vi "Main_old.vi"() -> ()   [LabVIEW 2020]
uses:
  States.ctl
  <vilib>/Instr/_visa.llb/VISA Configure Serial Port (Serial Instr).vi
  <vilib>/Utility/file.llb/Read Delimited Spreadsheet (I64).vi
panel:
  out "Last Inc Sent":string
  out "Last Speed Sent":string
  out "Next Control State":T1
  out "Next Com State":enum16{"Initialize", "Send", "Receive", "Error"}(ring)=enum."Receive"
  out "Next Cmd":enum16{"getParm", "inc", "mph", "err"}(ring)
  out "Send Buffer":string
  out "Control Error":errorcluster
  out "Com Error":errorcluster
  out "Missed Msg":u16
  out "Time Left":u32
  out "Inc Changed":bool
  out "Next MPH":u16
  out "Next Duration":u16
  out "Next Inc":u16
  out "PD READ":u8
  out "INC READ":u8
  out "MPH READ":u8
  out "dwell":u16[](array[numeric])
  out "incline":u16[](array[numeric])
  out "time":u16[](array[numeric])
  out "speed":u16[](array[numeric])
  out "input lines":i32
  in  "TestScript":path=path "C:/LabView Computer Backup SEAL2788/DonP_TRM500/FootTimeInc.txt"
  out "read buffer":string
  out "Speed Changed":bool
  in  "Manual Stop":bool
  in  "Serial Port":refnum<visa-resource-name>="COM8"
  out "FootPath":path
  out "FootPathRef":refnum<file>
  out "stopping":bool
  out "Target MPH":u16 max=12 step=1
  out "step":i32
  out "Target INC":u16 max=12 step=1
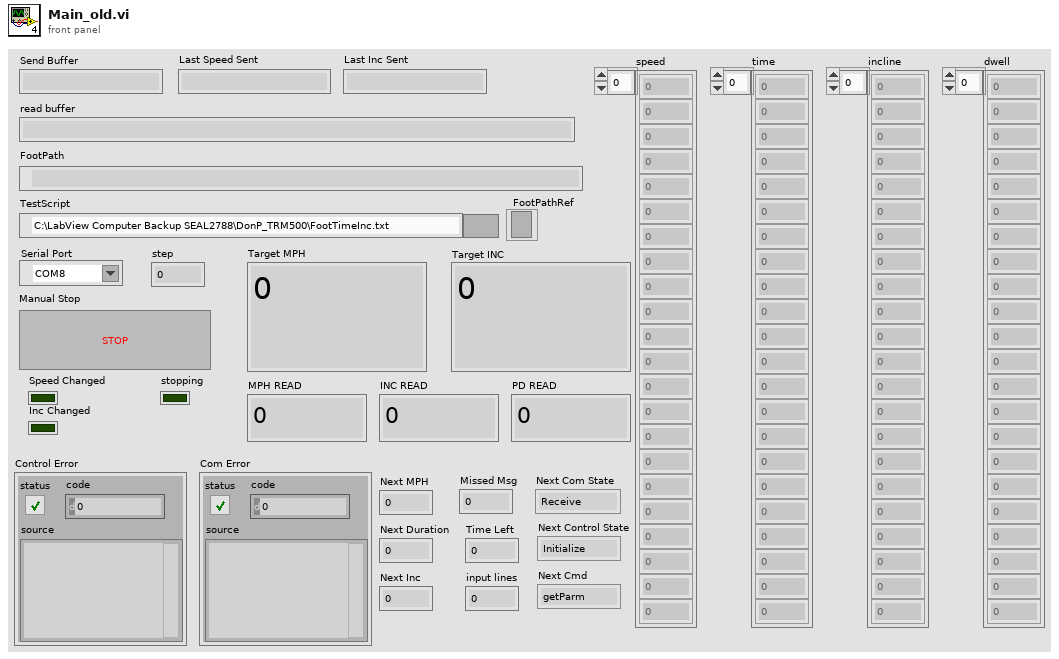
[diagram p1: front panel]
types:
  T1 = typedef "States.ctl" = enum16{"Initialize", "SetTargets", "WaitforMPH", "Dwell", "CheckTiming"}
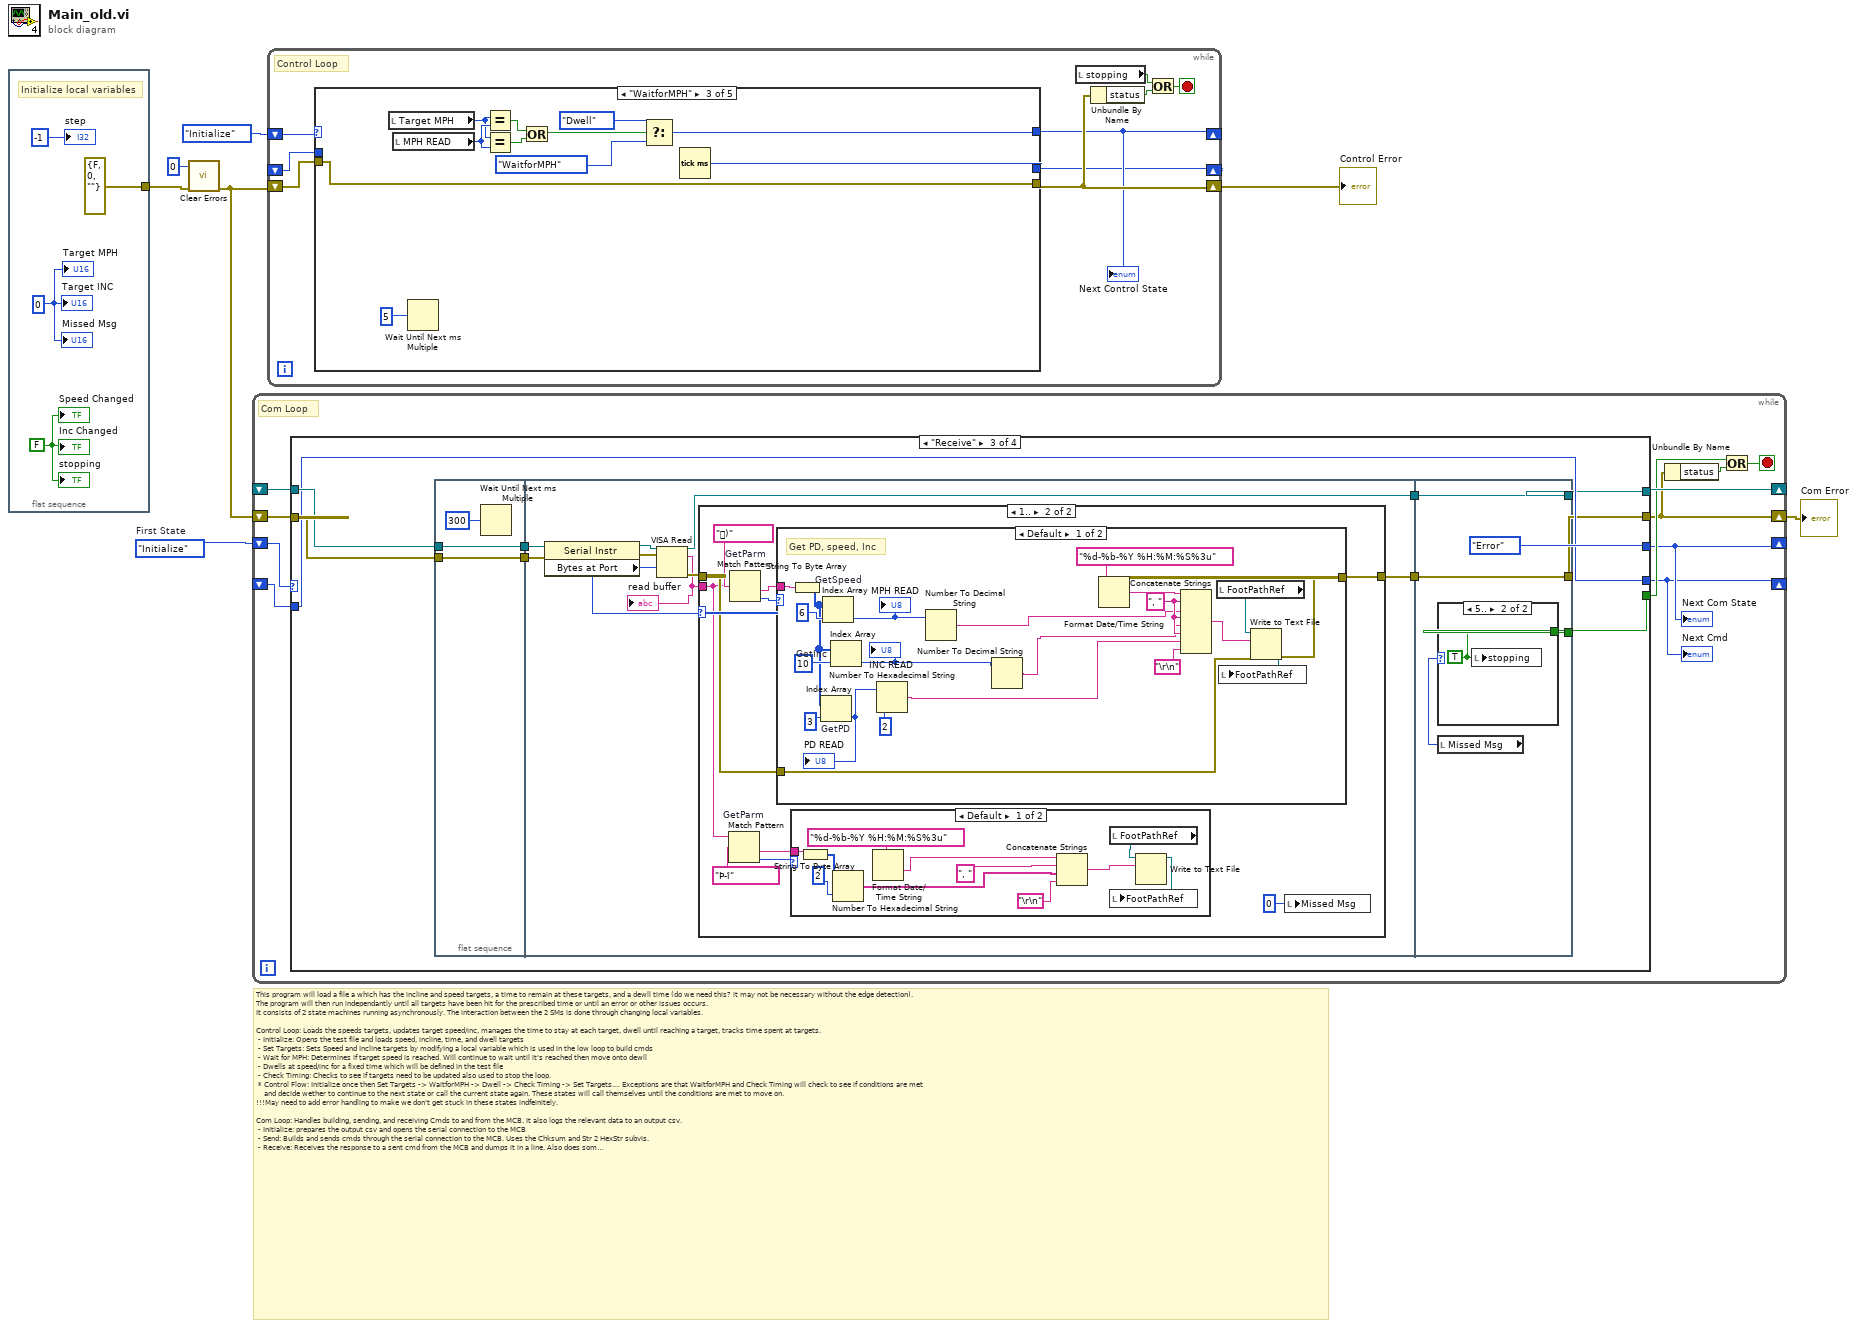
[diagram p0: block diagram]
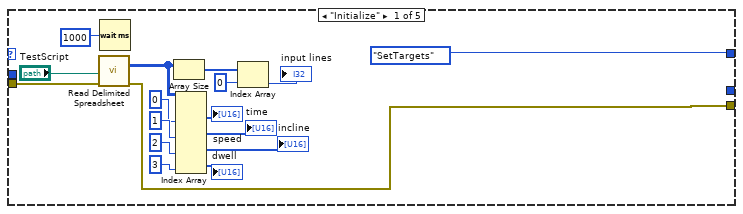
[diagram p2: hidden frame]
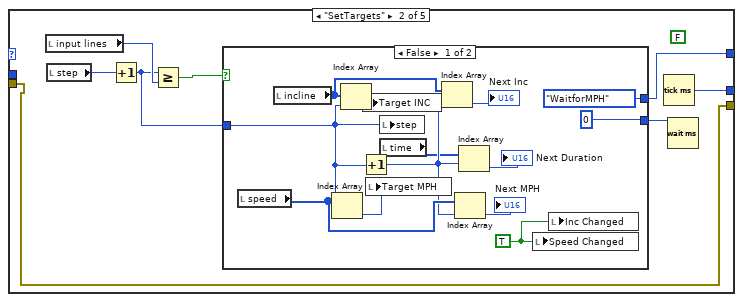
[diagram p3: hidden frame]
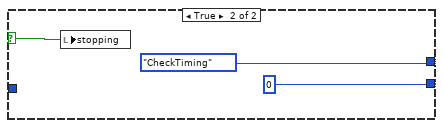
[diagram p4: hidden frame]
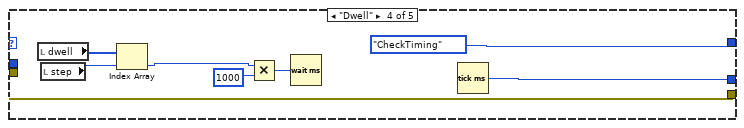
[diagram p5: hidden frame]
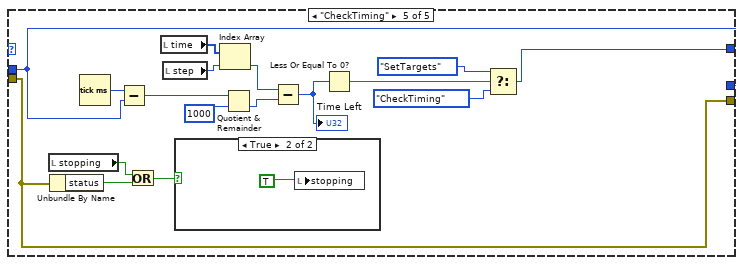
[diagram p6: hidden frame]
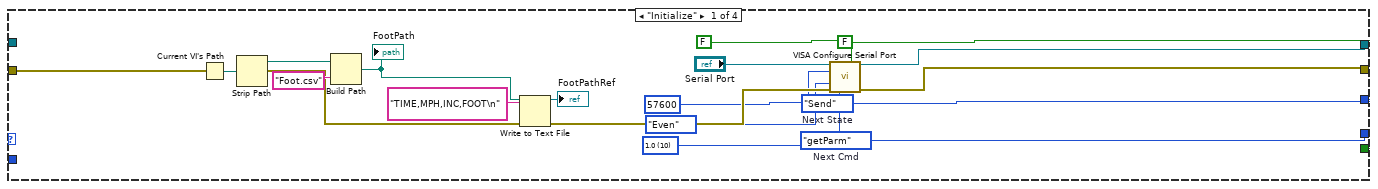
[diagram p8: hidden frame]
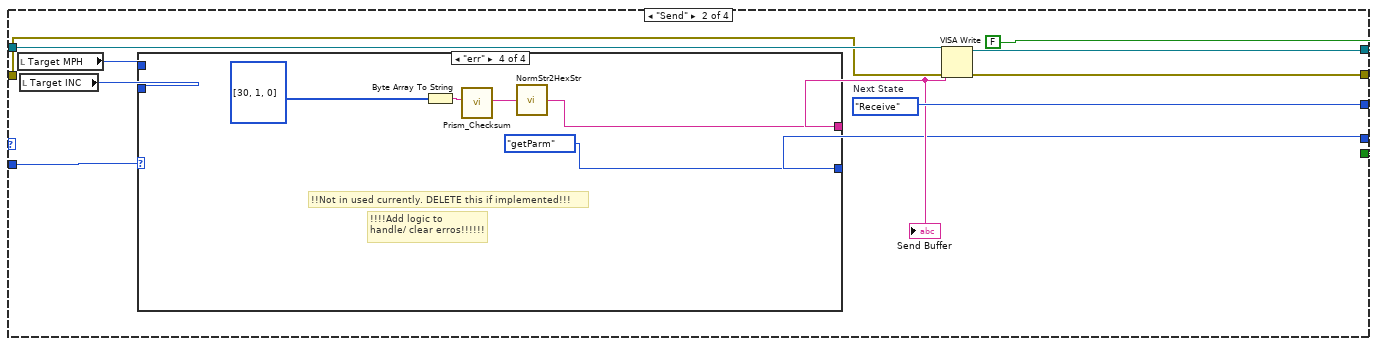
[diagram p9: hidden frame]
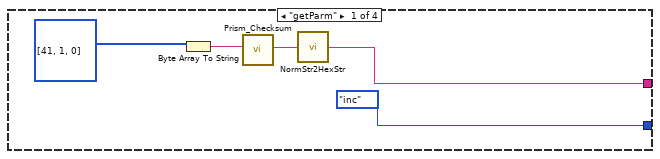
[diagram p10: hidden frame]
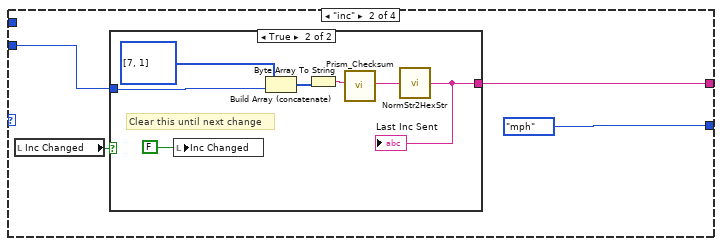
[diagram p11: hidden frame]
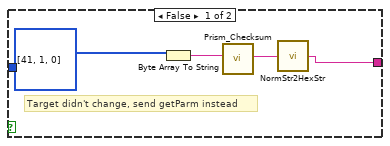
[diagram p12: hidden frame]
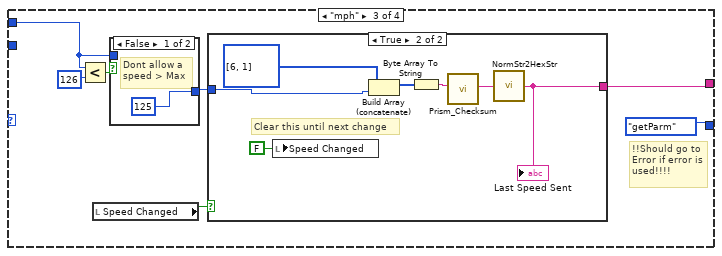
[diagram p13: hidden frame]
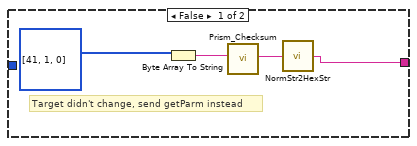
[diagram p15: hidden frame]
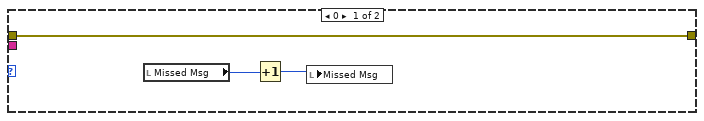
[diagram p16: hidden frame]
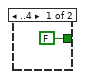
[diagram p19: hidden frame]
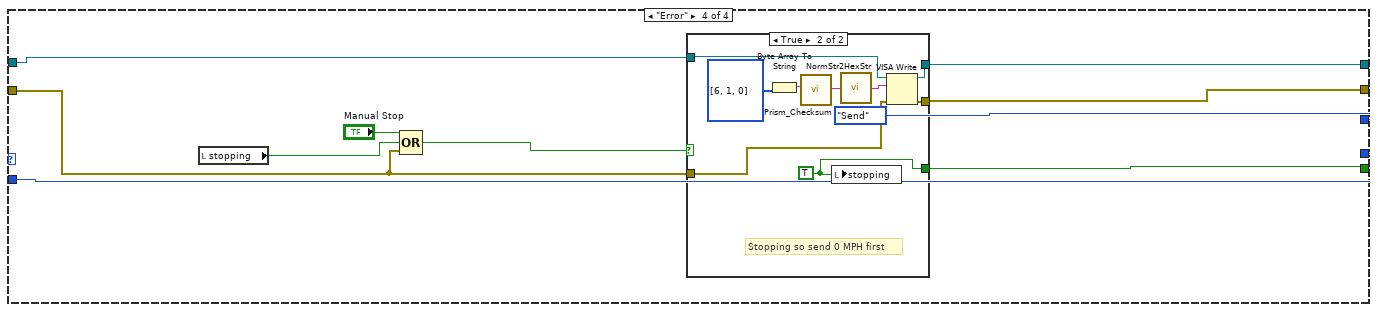
[diagram p20: hidden frame]
diagram:
  w7 = enum16{"Initialize", "Send", "Receive", "Error"}."Initialize"  # First State
  # "This program will load a file a which has the incline and speed targets, a time to remain at these targets, and a dewll time (do we need this? it may not be necessary without the edge detection).\nThe program will then run independantly until all targets have been hit for the prescribed time or until an error or other issues occurs.\nIt consists of 2 state machines running asynchronously. The interaction between the 2 SMs is done through changing local variables.\n\nControl Loop: Loads the speeds targets, updates target speed/inc, manages the time to stay at each target, dwell until reaching a target, tracks time spent at targets. \n - Initialize: Opens the test file and loads speed, incline, time, and dwell targets \n - Set Targets: Sets Speed and Incline targets by modifying a local variable which is used in the low loop to build cmds \n - Wait for MPH: Determines if target speed is reached. Will continue to wait until it's reached then move onto dewll\n - Dwells at speed/inc for a fixed time which will be defined in the test file\n - Check Timing: Checks to see if targets need to be updated also used to stop the loop.\n * Control Flow: Initialize once then Set Targets -> WaitforMPH -> Dwell -> Check Timing -> Set Targets.... Exceptions are that WaitforMPH and Check Timing will check to see if conditions are met\n    and decide wether to continue to the next state or call the current state again. These states will call themselves until the conditions are met to move on. \n!!!May need to add error handling to make we don't get stuck in these states indfeinitely.\n\nCom Loop: Handles building, sending, and receiving Cmds to and from the MCB. It also logs the relevant data to an output csv.\n - Initialize: prepares the output csv and opens the serial connection to the MCB\n - Send: Builds and sends cmds through the serial connection to the MCB. Uses the Chksum and Str 2 HexStr subvis. \n - Receive: Receives the response to a sent cmd from the MCB and dumps it in a line. Also does some analysis of the response to determine current  Speed/inc/person detect\n - Error:  Stops the program. This handles labview errors and will stop the program when one is encounted. It also handles stopping when reaching the end of a test \n * Com Flow: nitialize once then Send -> Receive -> Error -> Send...\n * Send flow: GetParm -> Inc -> MPH -> GetParm etc. Exception is that it will check first to see if the target changed and if it hasn't will send getParm Instead\n!!!May need to add error handling in which case the flow should be GetParm -> MPH -> Inc -> Err -> GetParm....\n\nFiles:\n1 input file which contains the test script to run. Format: Speed, Time, Inc, Dwell. Time = time to stay at target speed/inc. Dwell = a fixed time to wait after reaching targets and before starting the Time counter. This is used to make sure the speed stablizes before starting the Time counter.\n1 output file which contains Timestamp, Speed, Incline, and a flag for if person is detected (0 = No, 1 = Yes). Format: TIME,MPH,INC,FOOT"
  n1 = flat-sequence {
    tunnel: [errorcluster {"status"=FALSE, "code"=0, "source"=""} ("error constant")] -> w3
    frame #0 {
      w9 = FALSE ("Inc Changed")
      w8 = u16 0 ("MPH")
      # "Initialize local variables"
      "stopping" <- w9
      "Target MPH" <- w8
      "step" <- -1 ("step")
      "Target INC" <- w8
      "Speed Changed" <- w9
      "Inc Changed" <- w9
      "Missed Msg" <- w8
    }
  }
  n2 = call <vilib>:"Clear Errors.vi"("error in (no error)"=w3, "specific error code to clear (0: all)"=0) -> ("error out"=w2:errorcluster)  [unwired: 4 in, 1 out]
  n3 = while {
    shift-right: [w16] -> w6
    shift-left: w2 -> [w22]
    shift-right: [w19] -> _
    shift-left: _ -> [w21]
    shift-right: [w13] -> _
    shift-left: w7 -> [w20]
    shift-right: [w12] -> _
    shift-left: _ -> [w18]
    stop <- w15 stop-if-true
    # "Com Loop"
    n4 = case shown="\"Receive\"" w20 {
      tunnel: w22 -> [w28 w42 w105 w175]
      tunnel: w21 -> [_ w49 w107 w173]
      tunnel: [w38 w51 w101 w172] -> w19
      tunnel: [w37 w50 w100 w174] -> w16
      tunnel: [w34 w45 enum16{"Initialize", "Send", "Receive", "Error"}."Error" enum16{"Initialize", "Send", "Receive", "Error"}."Send"] -> w13
      tunnel: [w36 w43 w104 w180] -> w12
      tunnel: w18 -> [_ w41 w104 w180]
      tunnel: [FALSE FALSE w97 w176] -> w17
      frame "Initialize" {
        w23 = u16 10 items=["1.0"=10, "1.5"=15, "2.0"=20] ("stop bits (10: 1 bit)")
        w34 = enum16{"Initialize", "Send", "Receive", "Error"}."Send"  # Next State
        w36 = enum16{"getParm", "inc", "mph", "err"}."getParm"  # Next Cmd
        n5 = Current VI's Path() -> (path=w33:path)
        n6 = Strip Path(path=w33) -> (stripped path=w32:path)  [unwired: 1 out]
        n7 = Build Path(base path=w32, name or relative path="Foot.csv") -> (appended path=w29:path)
        "FootPath" <- w29
        n8 = Write to Text File(file (use dialog)=w29, text="TIME,MPH,INC,FOOT\n", error in=w28) -> (refnum out=→"FootPathRef":refnum<file>, error out=w27:errorcluster)  [unwired: 1 in, 1 out]
        n9 = call-poly "VISA Configure Serial Port"("VISA resource name"="Serial Port", "Enable Termination\nChar (T)"=FALSE ("Enable Termination\nChar (T)"), "baud rate (9600)"=u32 57600, "parity (0:none)"=enum16{"None", "Odd", "Even", "Mark", "Space"}."Even", "error in (no error)"=w27, "stop bits (10: 1 bit)"=w23) -> ("VISA resource name out"=w38:refnum<visa-resource-name>, "error out"=w37:errorcluster)  [unwired: 8 in]
      }
      frame "Send" {
        w45 = enum16{"Initialize", "Send", "Receive", "Error"}."Receive"  # Next State
        n10 = local read "Target MPH"() -> (w47:u16)
        n11 = local read "Target INC"() -> (w46:u16)
        n12 = case shown="\"err\"" w41 {
          tunnel: w47 -> [_ _ w73 _]
          tunnel: w46 -> [_ w60 _ _]
          tunnel: [w52 w59 w77 w93] -> w44
          tunnel: [enum16{"getParm", "inc", "mph", "err"}."inc" enum16{"getParm", "inc", "mph", "err"}."mph" enum16{"getParm", "inc", "mph", "err"}."getParm" enum16{"getParm", "inc", "mph", "err"}."getParm"] -> w43
          frame "getParm" {
            n13 = Byte Array To String(unsigned byte array=u8[] [41, 1, 0]) -> (string=w54:string)
            n14 = call "Prism_Checksum.vi"("ID +DB+ Data"=w54) -> ("Full Cmd"=w53:string)  [unwired: 10 in]
            n15 = call "NormStr2HexStr.vi"("string"=w53) -> ("hex string"=w52:string)
          }
          frame "inc" {
            n16 = local read "Inc Changed"() -> (w57:bool)
            n17 = case shown="True" w57 {
              tunnel: w60 -> [_ w68]
              tunnel: [w61 w66] -> w59
              frame False {
                # "Target didn't change, send getParm instead"
                n18 = Byte Array To String(unsigned byte array=u8[] [41, 1, 0]) -> (string=w63:string)
                n19 = call "Prism_Checksum.vi"("ID +DB+ Data"=w63) -> ("Full Cmd"=w62:string)  [unwired: 10 in]
                n20 = call "NormStr2HexStr.vi"("string"=w62) -> ("hex string"=w61:string)
              }
              frame True {
                # "Clear this until next change"
                n21 = local write "Inc Changed"(FALSE ("Value Changed")) -> ()
                n22 = Build Array (concatenate)(u8[] [7, 1] ("unsigned byte array"), w68) -> (w67:u16[])
                n23 = Byte Array To String(unsigned byte array=w67) -> (string=w70:string)
                n24 = call "Prism_Checksum.vi"("ID +DB+ Data"=w70) -> ("Full Cmd"=w71:string)  [unwired: 10 in]
                n25 = call "NormStr2HexStr.vi"("string"=w71) -> ("hex string"=w66:string)
                "Last Inc Sent" <- w66
              }
            }
          }
          frame "mph" {
            # "!!Should go to\nError if error is\nused!!!!"
            n26 = Less?(x=w73, y=u16 126) -> (x < y?=w75:bool)
            n27 = local read "Speed Changed"() -> (w76:bool)
            n28 = case shown="False" w75 {
              tunnel: w73 -> [_ w80]
              tunnel: [u16 125 ("Target MPH") w80] -> w72
              frame False {
                # "Dont allow a\nspeed > Max"
              }
              frame True {
              }
            }
            n29 = case shown="True" w76 {
              tunnel: [w81 w88] -> w77
              tunnel: w72 -> [_ w86]
              frame False {
                # "Target didn't change, send getParm instead"
                n30 = Byte Array To String(unsigned byte array=u8[] [41, 1, 0]) -> (string=w83:string)
                n31 = call "Prism_Checksum.vi"("ID +DB+ Data"=w83) -> ("Full Cmd"=w82:string)  [unwired: 10 in]
                n32 = call "NormStr2HexStr.vi"("string"=w82) -> ("hex string"=w81:string)
              }
              frame True {
                # "Clear this until next change"
                n33 = local write "Speed Changed"(FALSE ("Value Changed")) -> ()
                n34 = Build Array (concatenate)(u8[] [6, 1] ("unsigned byte array"), w86) -> (w87:u16[])
                n35 = Byte Array To String(unsigned byte array=w87) -> (string=w90:string)
                n36 = call "Prism_Checksum.vi"("ID +DB+ Data"=w90) -> ("Full Cmd"=w91:string)  [unwired: 10 in]
                n37 = call "NormStr2HexStr.vi"("string"=w91) -> ("hex string"=w88:string)
                "Last Speed Sent" <- w88
              }
            }
          }
          frame "err" {
            # "!!Not in used currently. DELETE this if implemented!!!"
            # "!!!!Add logic to\nhandle/ clear erros!!!!!!"
            n38 = Byte Array To String(unsigned byte array=u8[] [30, 1, 0]) -> (string=w95:string)
            n39 = call "Prism_Checksum.vi"("ID +DB+ Data"=w95) -> ("Full Cmd"=w96:string)  [unwired: 10 in]
            n40 = call "NormStr2HexStr.vi"("string"=w96) -> ("hex string"=w93:string)
          }
        }
        "Send Buffer" <- w44
        n41 = VISA Write(VISA resource name=w49, write buffer=w44, error in (no error)=w42) -> (VISA resource name out=w51:refnum<visa-resource-name>, error out=w50:errorcluster)  [unwired: 1 out]
      }
      frame "Receive" {
        n42 = flat-sequence {
          tunnel: w107 -> [w109]
          tunnel: w105 -> [w108]
          tunnel: [w109] -> w103
          tunnel: [w108] -> w102
          tunnel: w103 -> [w119]
          tunnel: w102 -> [w118]
          tunnel: [w111] -> w99
          tunnel: [w115] -> w98
          tunnel: [w168] -> w100
          tunnel: [w169] -> w101
          tunnel: w99 -> [w169]
          tunnel: w98 -> [w168]
          tunnel: [w166] -> w97
          frame #0 {
            n43 = Wait Until Next ms Multiple(millisecond multiple=u32 300) -> ()  [unwired: 1 out]
          }
          frame #1 {
            n44 = property class="Serial Instr"(reference=w119, error in=w118) -> (reference out=w116:refnum<visa-resource-name>, error out=w117:errorcluster, "Bytes at Port"=w114:u32)
            n45 = VISA Read(VISA resource name=w116, byte count=w114, error in (no error)=w117) -> (VISA resource name out=w111:refnum<visa-resource-name>, read buffer=w112:string, error out=w113:errorcluster)  [unwired: 1 out]
            "read buffer" <- w112
            n46 = case shown="1.." w114 {
              tunnel: [w122 w129] -> w115
              tunnel: w113 -> [w122 w128]
              tunnel: w112 -> [_ w127]
              frame 0 {
                n47 = local read "Missed Msg"() -> (w121:u16)
                n48 = Increment(x=w121) -> (x+1=w120:u16)
                n49 = local write "Missed Msg"(w120) -> ()
              }
              frame 1.. {
                n50 = Match Pattern "GetParm"(string=w127, regular expression="Þ­î") -> (after substring=w124:string, offset past match=w125:i32)  [unwired: 1 in, 2 out]
                n51 = Match Pattern "GetParm"(string=w127, regular expression="ޭ)") -> (after substring=w131:string, offset past match=w130:i32)  [unwired: 1 in, 2 out]
                n52 = case shown="Default" w130 {
                  tunnel: w131 -> [w145 _]
                  tunnel: [w158 w165] -> w129
                  tunnel: w128 -> [w153 w165]
                  frame Default {
                    w152 = ", "
                    # "Get PD, speed, Inc"
                    n53 = String To Byte Array(string=w145) -> (unsigned byte array=w161:u8[])
                    n54 = Index Array "GetPD"(array=w161, index=3) -> (element=w155:u8)
                    "PD READ" <- w155
                    n55 = Index Array "GetSpeed"(array=w161, index=6) -> (element=w147:u8)
                    "MPH READ" <- w147
                    n56 = Index Array "GetInc"(array=w161, index=10) -> (element=w146:u8)
                    "INC READ" <- w146
                    n57 = Number To Hexadecimal String(1:i16 2 ("width (-)"), 2:w155) -> (0:w150:string)
                    n58 = Number To Decimal String(number=w147) -> (decimal integer string=w149:string)  [unwired: 1 in]
                    n59 = Number To Decimal String(number=w146) -> (decimal integer string=w148:string)  [unwired: 1 in]
                    n60 = Format Date/Time String(time format string (%c)="%d-%b-%Y %H:%M:%S%3u") -> (date/time string=w156:string)  [unwired: 2 in]
                    n61 = Concatenate Strings(w156, w152, w149, w152, w148, w152, w150, "\r\n") -> (w159:string)
                    n62 = local read "FootPathRef"() -> (w157:refnum<file>)
                    n63 = Write to Text File(file (use dialog)=w157, text=w159, error in=w153) -> (refnum out=w151:refnum<file>, error out=w158:errorcluster)  [unwired: 1 in, 1 out]
                    n64 = local write "FootPathRef"(w151) -> ()
                  }
                  frame -1 {
                  }
                }
                n65 = case shown="Default" w125 {
                  tunnel: w124 -> [w138 _]
                  frame Default {
                    n66 = String To Byte Array(string=w138) -> (unsigned byte array=w136:u8[])
                    n67 = Number To Hexadecimal String(1:i16 2 ("width (-)"), 2:w136) -> (0:w133:string[])
                    n68 = Format Date/Time String(time format string (%c)="%d-%b-%Y %H:%M:%S%3u") -> (date/time string=w140:string)  [unwired: 2 in]
                    n69 = Concatenate Strings(w140, ", ", w133, "\r\n") -> (w139:string)
                    n70 = local read "FootPathRef"() -> (w143:refnum<file>)
                    n71 = Write to Text File(file (use dialog)=w143, text=w139) -> (refnum out=w142:refnum<file>)  [unwired: 2 in, 2 out]
                    n72 = local write "FootPathRef"(w142) -> ()
                  }
                  frame -1 {
                  }
                }
                n73 = local write "Missed Msg"(u16 0 ("Missed Msg")) -> ()
              }
            }
          }
          frame #2 {
            n74 = local read "Missed Msg"() -> (w167:u16)
            n75 = case shown="5.." w167 {
              tunnel: [FALSE ("stopping") w171] -> w166
              frame ..4 {
              }
              frame 5.. {
                w171 = TRUE ("stopping")
                n76 = local write "stopping"(w171) -> ()
              }
            }
          }
        }
      }
      frame "Error" {
        n77 = local read "stopping"() -> (w177:bool)
        n78 = Compound Arithmetic op=OR("Manual Stop", w177, w175) -> (w179:bool)
        n79 = case shown="True" w179 {
          tunnel: [FALSE w193] -> w176
          tunnel: w175 -> [w183 w188]
          tunnel: [w183 w187] -> w174
          tunnel: w173 -> [w182 w186]
          tunnel: [w182 w185] -> w172
          frame False {
          }
          frame True {
            w193 = TRUE ("stopping")
            # "Stopping so send 0 MPH first"
            n80 = Byte Array To String(unsigned byte array=u8[] [6, 1, 0]) -> (string=w192:string)
            n81 = call "Prism_Checksum.vi"("ID +DB+ Data"=w192) -> ("Full Cmd"=w191:string)  [unwired: 10 in]
            n82 = local write "stopping"(w193) -> ()
            n83 = call "NormStr2HexStr.vi"("string"=w191) -> ("hex string"=w190:string)
            n84 = VISA Write(VISA resource name=w186, write buffer=w190, error in (no error)=w188) -> (VISA resource name out=w185:refnum<visa-resource-name>, error out=w187:errorcluster)  [unwired: 1 out]
          }
        }
      }
    }
    "Next Com State" <- w13
    "Next Cmd" <- w12
    n85 = Unbundle By Name(w16) -> ("status"=w14:bool)
    n86 = Or(x=w17, y=w14) -> (x .or. y?=w15:bool)
  }
  "Com Error" <- w6
  n87 = while {
    shift-right: [w199] -> w5
    shift-left: w2 -> [w202]
    shift-right: [w197] -> _
    shift-left: _ -> [w196]
    shift-right: [w198] -> _
    shift-left: States."Initialize" ("First State") -> [w195]
    stop <- w200 stop-if-true
    # "Control Loop"
    n88 = case shown="\"WaitforMPH\"" w195 {
      tunnel: w202 -> [w217 w220 w253 w259 w263]
      tunnel: [w207 w220 w253 w259 w263] -> w199
      tunnel: [States."SetTargets" ("First State") w224 w251 States."CheckTiming" ("First State") w264] -> w198
      tunnel: [_ w222 w252 w256 w275] -> w197
      tunnel: w196 -> [_ _ _ _ w275]
      frame "Initialize" {
        n89 = call-poly <vilib>:"Read Delimited Spreadsheet.vi"("file path (dialog if empty)"="TestScript", "error in (no error)"=w217) -> ("all rows"=w213:i64[][], "error out"=w207:errorcluster)  [unwired: 8 in, 4 out]
        n90 = Wait (ms)(milliseconds to wait=u32 1000) -> ()  [unwired: 1 out]
        n91 = Array Size(array=w213) -> (size(s)=w215:i32[])
        n92 = Index Array(array=w213, index (col) #1=0 ("index"), index (col) #2=1 ("index (col)"), index (col) #3=2 ("index (col)"), index (col) #4=3 ("index (col)")) -> (element #1=→"speed":i64[], element #2=→"time":i64[], element #3=→"incline":i64[], element #4=→"dwell":i64[])  [unwired: 4 in]
        n93 = Index Array(array=w215, index=0) -> (element=→"input lines":i32)
      }
      frame "SetTargets" {
        (unwired) FALSE
        n94 = local read "input lines"() -> (w226:i32)
        n95 = local read "step"() -> (w227:i32)
        n96 = Increment(x=w227) -> (x+1=w221:i32)
        n97 = Greater Or Equal?(x=w221, y=w226) -> (x >= y?=w225:bool)
        n98 = case shown="False" w225 {
          selector: w225 -> [_ w243]
          tunnel: [States."WaitforMPH" ("First State") States."CheckTiming" ("First State")] -> w224
          tunnel: [u32 0 ("milliseconds to wait") u32 0 ("milliseconds to wait")] -> w223
          tunnel: w221 -> [w238 _]
          frame False {
            w229 = TRUE ("Value Changed")
            n99 = local read "speed"() -> (w237:u16[])
            n100 = local read "incline"() -> (w236:u16[])
            n101 = Index Array(array=w237, index=w238) -> (element=w240:u16)
            n102 = Index Array(array=w236, index=w238) -> (element=w239:u16)
            n103 = Increment(x=w238) -> (x+1=w235:i32)
            n104 = local write "Target INC"(w239) -> ()
            n105 = local write "Target MPH"(w240) -> ()
            n106 = local write "step"(w238) -> ()
            n107 = local read "time"() -> (w234:u16[])
            n108 = Index Array(array=w236, index=w235) -> (element=→"Next Inc":u16)
            n109 = Index Array(array=w237, index=w235) -> (element=→"Next MPH":u16)
            n110 = Index Array(array=w234, index=w235) -> (element=→"Next Duration":u16)
            n111 = local write "Speed Changed"(w229) -> ()
            n112 = local write "Inc Changed"(w229) -> ()
          }
          frame True {
            n113 = local write "stopping"(w243) -> ()
          }
        }
        n114 = Tick Count (ms)() -> (millisecond timer value=w222:u32)
        n115 = Wait (ms)(milliseconds to wait=w223) -> ()  [unwired: 1 out]
      }
      frame "WaitforMPH" {
        n116 = local read "Target MPH"() -> (w246:u16)
        n117 = local read "MPH READ"() -> (w247:u8)
        n118 = Wait Until Next ms Multiple(millisecond multiple=u32 5) -> ()  [unwired: 1 out]
        n119 = Equal?(x=w246, y=w247) -> (x = y?=w249:bool)
        n120 = Equal?(x=w246, y=w247) -> (x = y?=w248:bool)
        n121 = Or(x=w249, y=w248) -> (x .or. y?=w250:bool)
        n122 = Select(t=States."Dwell" ("First State"), s=w250, f=States."WaitforMPH" ("First State")) -> (s? t:f=w251:T1)
        n123 = Tick Count (ms)() -> (millisecond timer value=w252:u32)
      }
      frame "Dwell" {
        n124 = local read "dwell"() -> (w257:u16[])
        n125 = local read "step"() -> (w258:i32)
        n126 = Index Array(array=w257, index=w258) -> (element=w262:u16)
        n127 = Multiply(x=w262, y=u16 1000) -> (x*y=w260:u16)
        n128 = Wait (ms)(milliseconds to wait=w260) -> ()  [unwired: 1 out]
        n129 = Tick Count (ms)() -> (millisecond timer value=w256:u32)
      }
      frame "CheckTiming" {
        n130 = local read "stopping"() -> (w277:bool)
        n131 = Unbundle By Name(w263) -> ("status"=w278:bool)
        n132 = Tick Count (ms)() -> (millisecond timer value=w279:u32)
        n133 = Subtract(x=w279, y=w275) -> (x-y=w274:u32)
        n134 = Or(x=w277, y=w278) -> (x .or. y?=w276:bool)
        n135 = local read "time"() -> (w272:u16[])
        n136 = local read "step"() -> (w271:i32)
        n137 = case shown="True" w276 {
          frame False {
          }
          frame True {
            n138 = local write "stopping"(TRUE ("stopping")) -> ()
          }
        }
        n139 = Index Array(array=w272, index=w271) -> (element=w269:u16)
        n140 = Quotient & Remainder(x=w274, y=u32 1000) -> (floor(x/y)=w270:u32)  [unwired: 1 out]
        n141 = Subtract(x=w269, y=w270) -> (x-y=w268:u32)
        "Time Left" <- w268
        n142 = Less Or Equal To 0?(x=w268) -> (x <= 0?=w267:bool)
        n143 = Select(t=States."SetTargets" ("First State"), s=w267, f=States."CheckTiming" ("First State")) -> (s? t:f=w264:T1)
      }
    }
    "Next Control State" <- w198
    n144 = local read "stopping"() -> (w194:bool)
    n145 = Unbundle By Name(w199) -> ("status"=w201:bool)
    n146 = Or(x=w194, y=w201) -> (x .or. y?=w200:bool)
  }
  "Control Error" <- w5
